vi "ValidateFilterDTO.vi"(8 "error in (no error)":errorcluster, 11 "FilterDTOin":T2={"mode"="Mirror", "levelMin"="INFO", "levelMax"="INFO", "tagPrefix"=""}) -> (0 "error out":errorcluster, 3 "FilterDTOout":T2={"mode"="mirror", "levelMin"="INFO", "levelMax"="INFO", "tagPrefix"=""})   [LabVIEW 2026, in "Lumberjack.lvlib"]
doc: "Validates a FilterDTO's mode and level band.\nParses mode to FilterMode and levelMin/levelMax to Severity (an unknown name raises a descriptive error) and checks the band is well-formed; passes the DTO through when valid.\nLumberjack.lvlib, community (friend of Tests.lvlib)."
uses:
  Lumberjack.lvlib
  TypeDefs/ConfigDTO/FilterDTO.ctl
  TypeDefs/Severity.ctl
  <vilib>/Utility/Data Type/NI_Data Type.lvlib
panel:
  out "LevelMaxLocal":T1=enum."INFO"
  out "LevelMinLocal":T1=enum."INFO"
  # "Note:\nMin = Most Severe (Lowest Rank),\nMax = Least Severe (Highest Rank)"
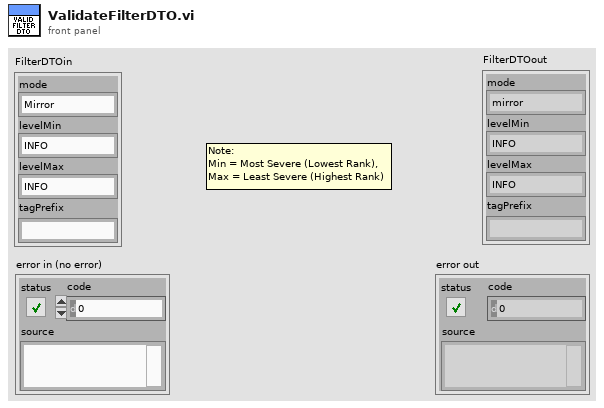
[diagram p1: front panel]
types:
  T1 = typedef "Lumberjack.lvlib/Severity.ctl" = enum16{"OFF", "FATAL", "ERROR", "WARN", "INFO", "DEBUG", "TRACE", "ALL"}
  T2 = typedef "Lumberjack.lvlib/FilterDTO.ctl" = cluster{"mode":string, "levelMin":string, "levelMax":string, "tagPrefix":string}
  T3 = typedef "NI_Data Type.lvlib/Data Type.ctl" = enum8{"Invalid Type", "Void", "I8", "I16", "I32", "I64", "U8", "U16", "U32", "U64", "Single Float", "Double Float", "Extended Float", "Single Complex", "Double Complex", "Extended Complex", "Enum U8", "Enum U16", "Enum U32", "Enum U64", "Single Float With Unit", "Double Float With Unit", "Extended Float With Unit", "Single Complex with Unit", "Double Complex with Unit", "Extended Complex with Unit", "Boolean", "String", "Path", "Picture", "Tag", "Array", "Cluster", "Variant", "LV Variant", "Waveform", "Timestamp", "Digital Waveform", "Digital Data", "ExpressData", "Refnum", "External Data", "VI", "Poly VI", "LabVIEW Class Instance", "Fixed Point", "Set Collection", "Map Collection"}
  T4 = typedef "NI_Data Type.lvlib/Type Definition Info.ctl" = cluster{"Name":string, "Timestamp":u32}
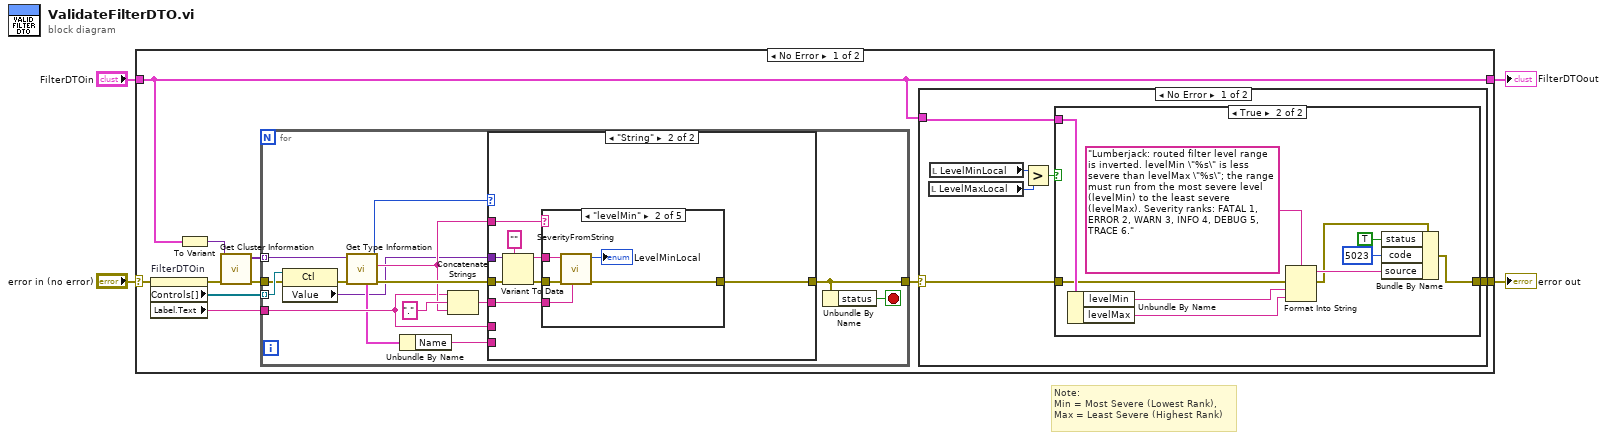
[diagram p0: block diagram]
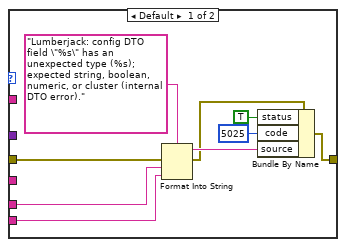
[diagram p4: hidden frame]
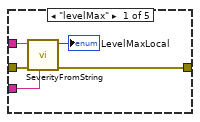
[diagram p5: hidden frame]
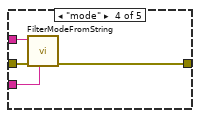
[diagram p7: hidden frame]
diagram:
  # "Note:\nMin = Most Severe (Lowest Rank),\nMax = Least Severe (Highest Rank)"
  n1 = case shown="No Error" "error in (no error)" {
    selector: "error in (no error)" -> [w8 w81]
    tunnel: "FilterDTOin" -> [w6 w82]
    tunnel: [w7 w81] -> w3
    tunnel: [w6 w82] -> w1
    frame No Error {
      n2 = property on="FilterDTOin" class="Clust (strict)"(error in=w8) -> (error out=w12:errorcluster, "Controls[]"=w9:refnum<vi>[], "Label.Text"=w10:string)  [unwired: 1 in, 1 out]
      n3 = To Variant(anything=w6) -> (Variant=w11:variant)
      n4 = call <vilib>:"Get Cluster Information.vi"("error in (no error)"=w12, "variant"=w11) -> ("error out"=w13:errorcluster, "cluster elements"=w14:variant[])  [unwired: 8 in]
      n5 = for {
        tunnel: w14 -> [w42] mode=indexing
        tunnel: w13 -> [w35]
        tunnel: w10 -> [w41]
        tunnel: [w38] -> w5
        tunnel: w9 -> [w36] mode=indexing
        stop <- w37 stop-if-true
        n6 = property class="Ctl"(reference=w36, error in=w35) -> (error out=w33:errorcluster, "Value"=w34:variant)  [unwired: 1 out]
        n7 = call <vilib>:"Get Type Information.vi"("error in (no error)"=w33, "variant"=w42) -> ("error out"=w46:errorcluster, "name"=w43:string, "type"=w44:T3, "type definition info"=w40:T4)  [unwired: 5 in, 1 out]
        n8 = Unbundle By Name(w40) -> ("Name"=w39:string)
        n9 = Concatenate Strings(w41, "." ("string"), w43) -> (w45:string)
        n10 = case shown="\"String\"" w44 {
          tunnel: w46 -> [w51 w62]
          tunnel: w45 -> [_ w64]
          tunnel: w43 -> [_ w63]
          tunnel: w34 -> [_ w60]
          tunnel: w41 -> [w52 _]
          tunnel: [w48 w57] -> w38
          tunnel: w39 -> [w49 _]
          frame Default {
            n11 = Format Into String(format string="Lumberjack: config DTO field \"%s\" has an unexpected type (%s); expected string, boolean, numeric, or cluster (internal DTO error)." ("source"), error in=w51, w52, w49) -> (resulting string=w56:string, error out=w50:errorcluster)  [unwired: 1 in]
            n12 = Bundle By Name(cluster=w50, "status"=TRUE, "code"=5025, "source"=w56) -> (w48:errorcluster)
          }
          frame "String" {
            n13 = Variant To Data(error in=w62, type="", Variant=w60) -> (data=w58:string, error out=w61:errorcluster)
            n14 = case shown="\"levelMin\"" w63 {
              tunnel: w61 -> [w69 w74 w75 w79 w80]
              tunnel: w64 -> [w68 w73 _ w78 _]
              tunnel: w58 -> [w67 w72 _ w77 _]
              tunnel: [w66 w71 w75 w76 w80] -> w57
              frame "levelMax" {
                n15 = call "SeverityFromString.vi"("Context"=w68, "error in (no error)"=w69, "SeverityString"=w67) -> ("error out"=w66:errorcluster, "Severity"=→"LevelMaxLocal":T1)  [unwired: 7 in]
              }
              frame "levelMin" {
                n16 = call "SeverityFromString.vi"("Context"=w73, "error in (no error)"=w74, "SeverityString"=w72) -> ("error out"=w71:errorcluster, "Severity"=→"LevelMinLocal":T1)  [unwired: 7 in]
              }
              frame "tagPrefix" {
              }
              frame "mode" {
                n17 = call "FilterModeFromString.vi"("Context"=w78, "error in (no error)"=w79, "FilterModeString"=w77) -> ("error out"=w76:errorcluster)  [unwired: 7 in, 1 out]
              }
              frame Default {
              }
            }
          }
        }
        n18 = Unbundle By Name(w38) -> ("status"=w37:bool)
      }
      n19 = case shown="No Error" w5 {
        selector: w5 -> [w18 w32]
        tunnel: [w20 w32] -> w7
        tunnel: w6 -> [w19 _]
        frame No Error {
          n20 = local read "LevelMaxLocal"() -> (w17:T1)
          n21 = local read "LevelMinLocal"() -> (w16:T1)
          n22 = Greater?(x=w16, y=w17) -> (0:w15:bool)
          n23 = case shown="True" w15 {
            tunnel: [w21 w26] -> w20
            tunnel: w19 -> [_ w25]
            tunnel: w18 -> [w21 w22]
            frame False {
            }
            frame True {
              n24 = Unbundle By Name(w25) -> ("levelMin"=w24:string, "levelMax"=w23:string)
              n25 = Format Into String(format string="Lumberjack: routed filter level range is inverted. levelMin \"%s\" is less severe than levelMax \"%s\"; the range must run from the most severe level (levelMin) to the least severe (levelMax). Severity ranks: FATAL 1, ERROR 2, WARN 3, INFO 4, DEBUG 5, TRACE 6." ("source"), error in=w22, w24, w23) -> (resulting string=w31:string, error out=w27:errorcluster)  [unwired: 1 in]
              n26 = Bundle By Name(cluster=w27, "status"=TRUE, "code"=5023, "source"=w31) -> (w26:errorcluster)
            }
          }
        }
        frame Error {
        }
      }
    }
    frame Error {
    }
  }
  "FilterDTOout" <- w1
  "error out" <- w3
